vi "get all names.vi"(8 "error in (no error)":errorcluster, 11 "SysObj in":refnum<class "system object.lvclass">) -> (0 "error out":errorcluster, 2 "Names":path[](array[path]), 3 "SysObj out":refnum<class "system object.lvclass">)   [LabVIEW 2020, in "system object.lvclass"]
uses:
  system object.lvclass
  system object.lvclass/system object.ctl
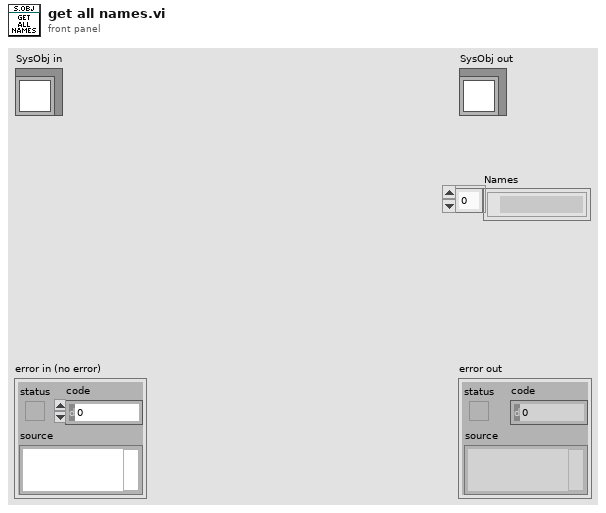
[diagram p1: front panel]
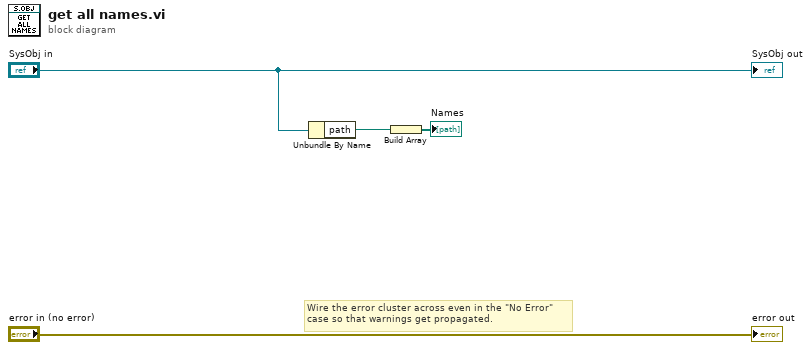
[diagram p0: block diagram]
diagram:
  # "Wire the error cluster across even in the \"No Error\"\ncase so that warnings get propagated."
  n1 = Unbundle By Name("SysObj in") -> ("path"=w2:path)
  n2 = Build Array(w2) -> (→"Names":path[])
  "error out" <- "error in (no error)"
  "SysObj out" <- "SysObj in"
